vi "Delete Helper.vi"(8 "error in (no error)":errorcluster, 9 "last key":string, 10 "Array":string[](array[string]), 11 "JSON Value in":refnum<class "JSON Value.lvclass">) -> (0 "error out":errorcluster, 3 "JSON Value out":refnum<class "JSON Value.lvclass">)   [LabVIEW 2016, in "JSON Value.lvclass"]
uses:
  JSON Value.lvclass
  JSON Value.lvclass/JSON Value.ctl
  New JSON Value/New JSON (Null).vi
  New JSON Value/New JSON ({}).vi
  Array/Delete/Delete from Array (Value).vi
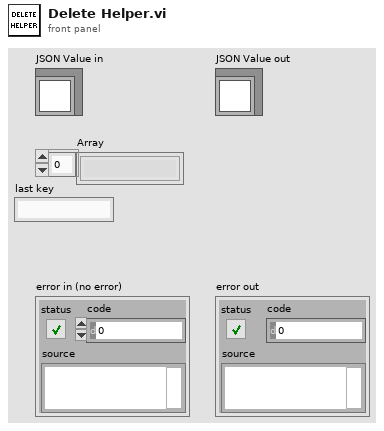
[diagram p1: front panel]
types:
  T1 = typedef "JSON Value.lvclass/JSON Types.ctl" = enum16{"String", "Numeric", "Boolean", "NULL", "Object", "Array"}
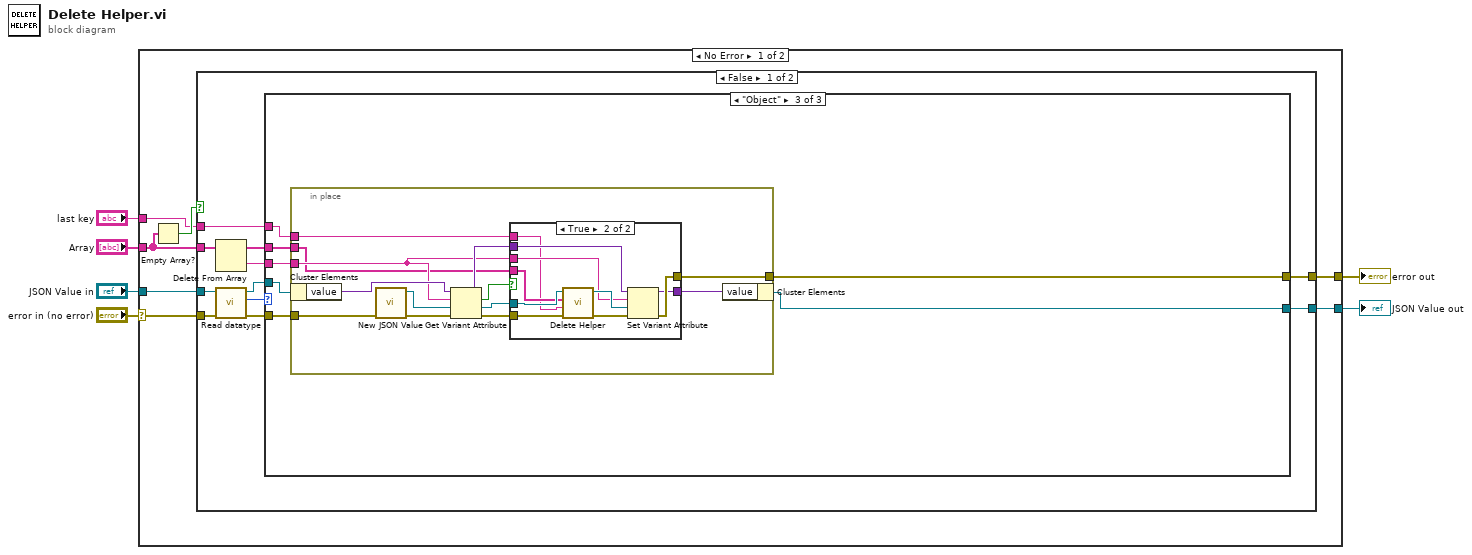
[diagram p0: block diagram]
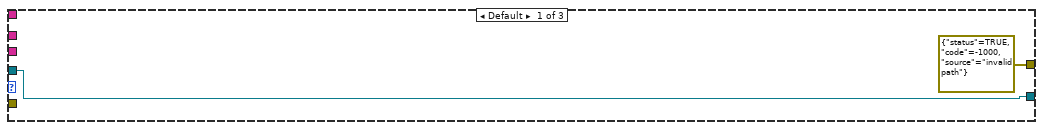
[diagram p2: hidden frame]
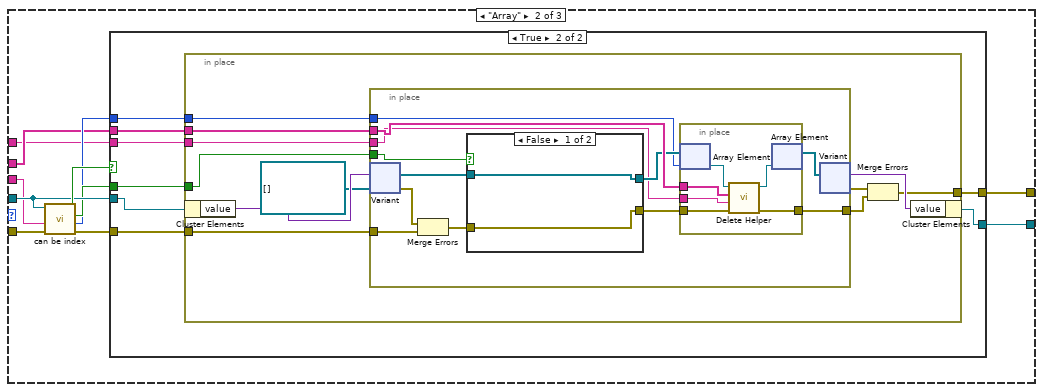
[diagram p3: hidden frame]
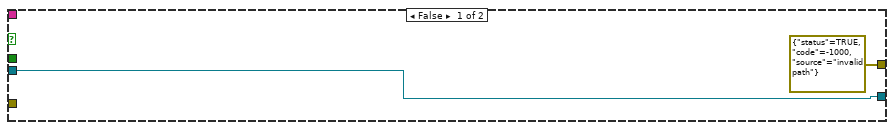
[diagram p4: hidden frame]
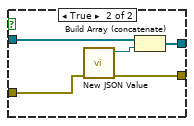
[diagram p5: hidden frame]
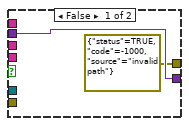
[diagram p6: hidden frame]
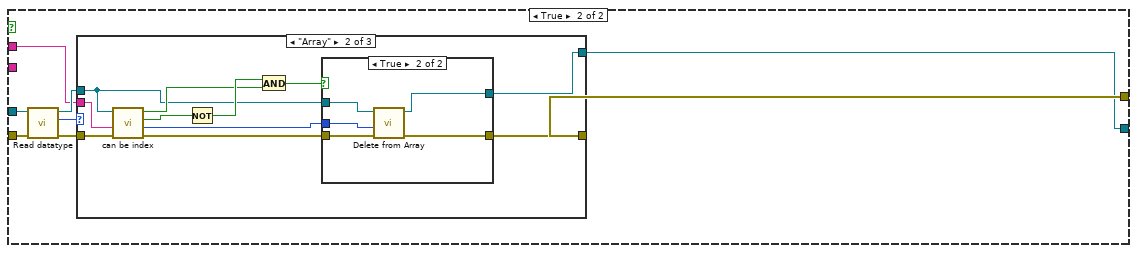
[diagram p7: hidden frame]
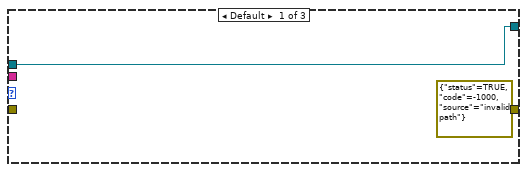
[diagram p8: hidden frame]
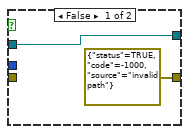
[diagram p9: hidden frame]
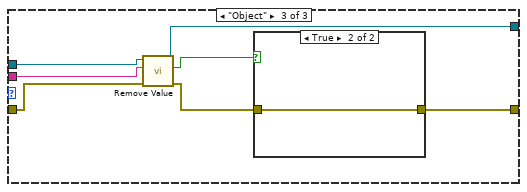
[diagram p10: hidden frame]
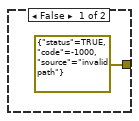
[diagram p11: hidden frame]
diagram:
  n1 = case shown="No Error" "error in (no error)" {
    selector: "error in (no error)" -> [w13 w154]
    tunnel: "JSON Value in" -> [w12 w153]
    tunnel: "Array" -> [w8 _]
    tunnel: [w11 w153] -> w3
    tunnel: [w10 w154] -> w2
    tunnel: "last key" -> [w7 _]
    frame No Error {
      n2 = Empty Array?(array=w8) -> (empty?=w9:bool)
      n3 = case shown="False" w9 {
        tunnel: w13 -> [w24 w123]
        tunnel: w12 -> [w21 w122]
        tunnel: [w19 w116] -> w11
        tunnel: [w18 w117] -> w10
        tunnel: w8 -> [w15 _]
        tunnel: w7 -> [w14 w119]
        frame False {
          n4 = Delete From Array(array=w15) -> (deleted portion=w16:string, array with subset deleted=w17:string[])  [unwired: 2 in]
          n5 = call "Read datatype.vi"("error in (no error)"=w24, "JSON Value in"=w21) -> ("error out"=w20:errorcluster, "datatype"=w23:T1, "JSON Value out"=w22:refnum<class "JSON Value.lvclass">)  [unwired: 7 in]
          n6 = case shown="\"Object\"" w23 {
            tunnel: w22 -> [w26 w36 w90]
            tunnel: w20 -> [_ w34 w89]
            tunnel: [w26 w33 w88] -> w19
            tunnel: [errorcluster {"status"=TRUE, "code"=-1000, "source"="invalid path"} ("error out") w30 w87] -> w18
            tunnel: w17 -> [_ w29 w85]
            tunnel: w16 -> [_ w28 w86]
            tunnel: w14 -> [_ w27 w84]
            frame Default {
            }
            frame "Array" {
              n7 = call "can be index.vi"("error in (no error)"=w34, "string"=w28, "JSON Value in"=w36) -> ("error out"=w35:errorcluster, "index"=w31:i32, "last value?"=w32:bool, "valid index?"=w37:bool)  [unwired: 5 in]
              n8 = case shown="True" w37 {
                tunnel: w36 -> [w39 w47]
                tunnel: w29 -> [_ w46]
                tunnel: w35 -> [_ w45]
                tunnel: [w39 w44] -> w33
                tunnel: w32 -> [_ w43]
                tunnel: w31 -> [_ w42]
                tunnel: [errorcluster {"status"=TRUE, "code"=-1000, "source"="invalid path"} ("error IO") w41] -> w30
                tunnel: w27 -> [_ w40]
                frame False {
                }
                frame True {
                  n9 = in-place {
                    in-place-border: w46 -> [w56]
                    in-place-border: w45 -> [w55]
                    in-place-border: w43 -> [w53]
                    in-place-border: w42 -> [w52]
                    in-place-border: [w49] -> w41
                    in-place-border: w40 -> [w48]
                    n10 = in-place-cluster #1(w47) -> ("value"=w58:variant)
                    n11 = in-place {
                      in-place-border: w56 -> [w70]
                      in-place-border: w55 -> [w63]
                      in-place-border: w53 -> [w68]
                      in-place-border: w52 -> [w65]
                      in-place-border: [w60] -> w51
                      in-place-border: w48 -> [w59]
                      n12 = in-place-variant #2(w58, refnum<class "JSON Value.lvclass">[] [] ("JSON Value out")) -> (w67:refnum<class "JSON Value.lvclass">[], w64:errorcluster)
                      n13 = Merge Errors(w64, w63) -> (w62:errorcluster)
                      n14 = case shown="False" w68 {
                        tunnel: w67 -> [w72 w77]
                        tunnel: [w72 w75] -> w66
                        tunnel: w62 -> [w71 w74]
                        tunnel: [w71 w73] -> w61
                        frame False {
                        }
                        frame True {
                          n15 = call-poly "New JSON Value.vi"("error in (no error)"=w74) -> ("error out"=w73:errorcluster, "JSON Value out"=w76:refnum<class "JSON Value.lvclass">)  [unwired: 9 in]
                          n16 = Build Array (concatenate)(w77, w76) -> (w75:refnum<class "JSON Value.lvclass">[])
                        }
                      }
                      n17 = in-place {
                        in-place-border: w70 -> [w81]
                        in-place-border: w61 -> [w80]
                        in-place-border: [w79] -> w60
                        in-place-border: w59 -> [w78]
                        n18 = in-place-array #3(w66, w65) -> (w83:refnum<class "JSON Value.lvclass">)
                        n19 = call "Delete Helper.vi"("error in (no error)"=w80, "last key"=w78, "Array"=w81, "JSON Value in"=w83) -> ("error out"=w79:errorcluster, "JSON Value out"=w82:refnum<class "JSON Value.lvclass">)  [unwired: 6 in]
                        n20 = in-place-array #3(w82) -> (w69:refnum<class "JSON Value.lvclass">[])  [unwired: 1 out]
                      }
                      n21 = in-place-variant #2(w69) -> (w54:variant, w50:errorcluster)
                    }
                    n22 = Merge Errors(w50, w51) -> (w49:errorcluster)
                    n23 = in-place-cluster #1("value"=w54) -> (w44:refnum<class "JSON Value.lvclass">)
                  }
                }
              }
            }
            frame "Object" {
              n24 = in-place {
                in-place-border: w85 -> [w98]
                in-place-border: w89 -> [w97]
                in-place-border: [w94] -> w87
                in-place-border: w86 -> [w99]
                in-place-border: w84 -> [w91]
                n25 = in-place-cluster #4(w90) -> ("value"=w103:variant)
                n26 = call-poly "New JSON Value.vi"("error in (no error)"=w97) -> ("error out"=w96:errorcluster, "JSON Value out"=w102:refnum<class "JSON Value.lvclass">)  [unwired: 9 in]
                n27 = Get Variant Attribute(Variant=w103, name=w99, default value (empty Variant)=w102, error in=w96) -> (duplicate Variant=w101:variant, found=w92:bool, value=w100:refnum<class "JSON Value.lvclass">, error out=w95:errorcluster)
                n28 = case shown="True" w92 {
                  tunnel: w101 -> [w105 w115]
                  tunnel: w100 -> [_ w114]
                  tunnel: w99 -> [_ w112]
                  tunnel: w98 -> [_ w111]
                  tunnel: w95 -> [_ w110]
                  tunnel: [errorcluster {"status"=TRUE, "code"=-1000, "source"="invalid path"} ("error out") w108] -> w94
                  tunnel: [w105 w107] -> w93
                  tunnel: w91 -> [_ w106]
                  frame False {
                  }
                  frame True {
                    n29 = call "Delete Helper.vi"("error in (no error)"=w110, "last key"=w106, "Array"=w111, "JSON Value in"=w114) -> ("error out"=w109:errorcluster, "JSON Value out"=w113:refnum<class "JSON Value.lvclass">)  [unwired: 6 in]
                    n30 = Set Variant Attribute(Variant=w115, name=w112, value=w113, error in=w109) -> (Variant out=w107:variant, error out=w108:errorcluster)  [unwired: 1 out]
                  }
                }
                n31 = in-place-cluster #4("value"=w93) -> (w88:refnum<class "JSON Value.lvclass">)
              }
            }
          }
        }
        frame True {
          n32 = call "Read datatype.vi"("error in (no error)"=w123, "JSON Value in"=w122) -> ("error out"=w118:errorcluster, "datatype"=w121:T1, "JSON Value out"=w120:refnum<class "JSON Value.lvclass">)  [unwired: 7 in]
          n33 = case shown="\"Array\"" w121 {
            tunnel: w120 -> [w124 w129 w146]
            tunnel: w119 -> [_ w136 w144]
            tunnel: w118 -> [_ w135 w148]
            tunnel: [errorcluster {"status"=TRUE, "code"=-1000, "source"="invalid path"} ("error out") w127 w150] -> w117
            tunnel: [w124 w126 w145] -> w116
            frame Default {
            }
            frame "Array" {
              n34 = call "can be index.vi"("error in (no error)"=w135, "string"=w136, "JSON Value in"=w129) -> ("error out"=w128:errorcluster, "index"=w130:i32, "last value?"=w134:bool, "valid index?"=w132:bool)  [unwired: 5 in]
              n35 = Not(x=w134) -> (.not. x?=w133:bool)
              n36 = And(x=w133, y=w132) -> (x .and. y?=w131:bool)
              n37 = case shown="True" w131 {
                tunnel: w130 -> [_ w142]
                tunnel: w129 -> [w137 w143]
                tunnel: w128 -> [_ w141]
                tunnel: [errorcluster {"status"=TRUE, "code"=-1000, "source"="invalid path"} ("error out") w140] -> w127
                tunnel: [w137 w139] -> w126
                frame False {
                }
                frame True {
                  n38 = call-poly "Delete from Array.vi"("error in (no error)"=w141, "index"=w142, "JSON Value in"=w143) -> ("error out"=w140:errorcluster, "JSON Value out"=w139:refnum<class "JSON Value.lvclass">)  [unwired: 6 in, 1 out]
                }
              }
            }
            frame "Object" {
              n39 = call "Remove Value.vi"("error in (no error)"=w148, "key"=w144, "JSON Value in"=w146) -> ("error out"=w147:errorcluster, "found"=w149:bool, "JSON Value out"=w145:refnum<class "JSON Value.lvclass">)  [unwired: 6 in]
              n40 = case shown="True" w149 {
                tunnel: w147 -> [_ w152]
                tunnel: [errorcluster {"status"=TRUE, "code"=-1000, "source"="invalid path"} ("error out") w152] -> w150
                frame False {
                }
                frame True {
                }
              }
            }
          }
        }
      }
    }
    frame Error {
    }
  }
  "JSON Value out" <- w3
  "error out" <- w2
